vi "Center of Circle.vi"(8 "Sign":dbl=-1.0, 9 "Tangent Point":cluster{dbl, dbl}, 10 "Tangent Angle":dbl, 11 "Radius":dbl) -> (3 "Center Point":cluster{dbl, dbl})   [LabVIEW 2018]
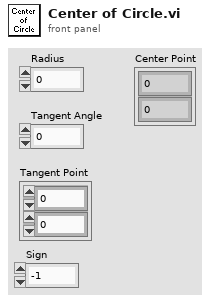
[diagram p1: front panel]
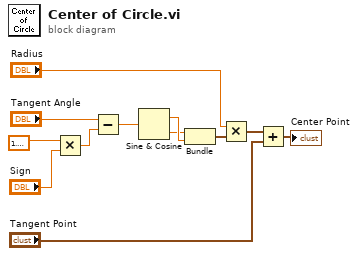
[diagram p0: block diagram]
diagram:
  n1 = Multiply(x=1.5707963267948966, y="Sign") -> (x*y=w2:dbl)
  n2 = Subtract(x="Tangent Angle", y=w2) -> (x-y=w5:dbl)
  n3 = Sine & Cosine(0:w5) -> (1:w7:dbl, 2:w6:dbl)
  n4 = Bundle(w6, w7) -> (w8:cluster{dbl, dbl})  [unwired: 1 in]
  n5 = Multiply(x="Radius", y=w8) -> (x*y=w9:cluster{dbl, dbl})
  n6 = Add(x=w9, y="Tangent Point") -> (x+y=→"Center Point":cluster{dbl, dbl})
